vi "OFDM_TransimitPreparation - 2 Channels.vi"(10 "array 2":cdb[](array[numeric]), 11 "array":cdb[](array[numeric])) -> (1 "2D array":cdb[][](array[numeric]), 2 "output array 2":cdb[](array[numeric]), 3 "output array":cdb[](array[numeric]))   [LabVIEW 2022 SP3]
panel:
  out "size(s) 2":i32
  out "size(s)":i32
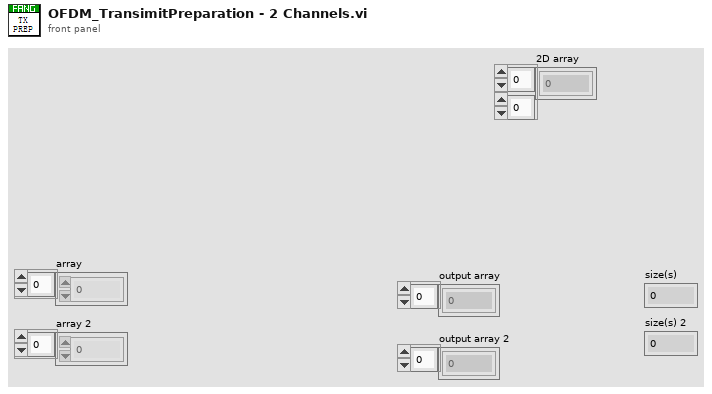
[diagram p1: front panel]
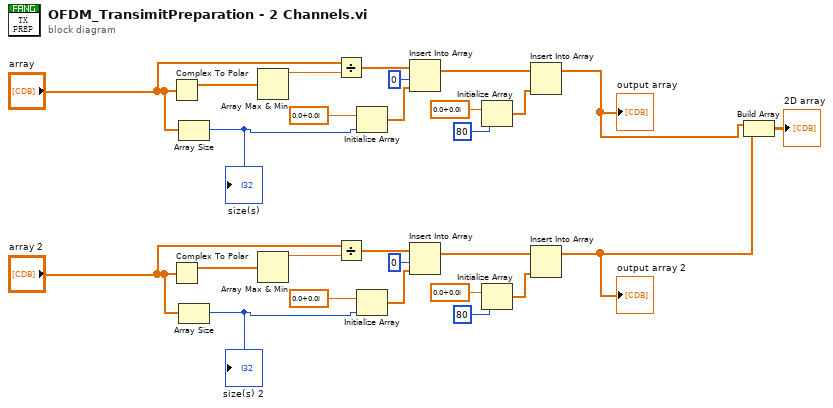
[diagram p0: block diagram]
diagram:
  n1 = Complex To Polar(r * e^(i*theta)="array") -> (r=w27:dbl[])  [unwired: 1 out]
  n2 = Complex To Polar(r * e^(i*theta)="array 2") -> (r=w15:dbl[])  [unwired: 1 out]
  n3 = Array Size(array="array") -> (size(s)=w16:i32)
  "size(s)" <- w16
  n4 = Array Size(array="array 2") -> (size(s)=w4:i32)
  "size(s) 2" <- w4
  n5 = Array Max & Min(array=w27) -> (max value=w26:dbl)  [unwired: 3 out]
  n6 = Array Max & Min(array=w15) -> (max value=w14:dbl)  [unwired: 3 out]
  n7 = Divide(x="array", y=w26) -> (x/y=w25:cdb[])
  n8 = Divide(x="array 2", y=w14) -> (x/y=w13:cdb[])
  n9 = Initialize Array(cdb 0.0+0.0i ("element"), w16) -> (w21:cdb[])
  n10 = Initialize Array(cdb 0.0+0.0i ("element"), w4) -> (w9:cdb[])
  n11 = Insert Into Array(array=w25, index=0, new element=w21) -> (w22:cdb[])
  n12 = Insert Into Array(array=w13, index=0, new element=w9) -> (w10:cdb[])
  n13 = Initialize Array(cdb 0.0+0.0i ("element"), 80 ("dimension size")) -> (w19:cdb[])
  n14 = Initialize Array(cdb 0.0+0.0i ("element"), 80 ("dimension size")) -> (w7:cdb[])
  n15 = Insert Into Array(array=w22, new element=w19) -> (w3:cdb[])  [unwired: 1 in]
  "output array" <- w3
  n16 = Insert Into Array(array=w10, new element=w7) -> (w2:cdb[])  [unwired: 1 in]
  "output array 2" <- w2
  n17 = Build Array(w3, w2) -> (→"2D array":cdb[][])
